vi "PNA_SHEET_DISPLAY.vi"(4 "Mode":i32(ring) items=["OFF", "ON"], 6 "SHEET":i32=1, 8 "error in (no error)":errorcluster, 11 "VISA resource name":refnum<visa-resource-name>) -> (0 "error out":errorcluster, 3 "VISA resource name out":refnum<visa-resource-name>)   [LabVIEW 2018, in "Agilent ENA Series.lvlib"]
doc: "Changes the state of each channel of selected channel to the startup state in the trigger system.\n\nWhen this function is executed for a channel in the idle state, it goes into the initiate state immediately. Then, after measurement is executed once, it goes back to the idle state.\n\nIf this function is executed for a channel that is not in the idle state or for which the continuous initiation mode is enabled, an error occurs."
uses:
  Agilent ENA Series.lvlib
panel:
  out "cmd":string
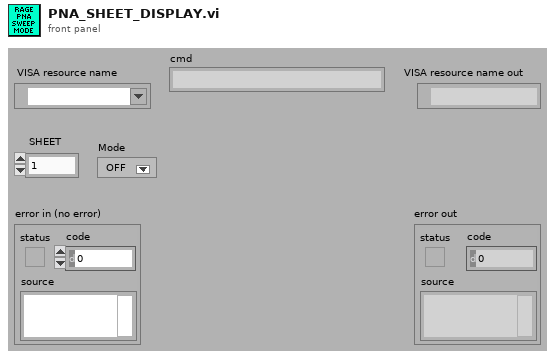
[diagram p1: front panel]
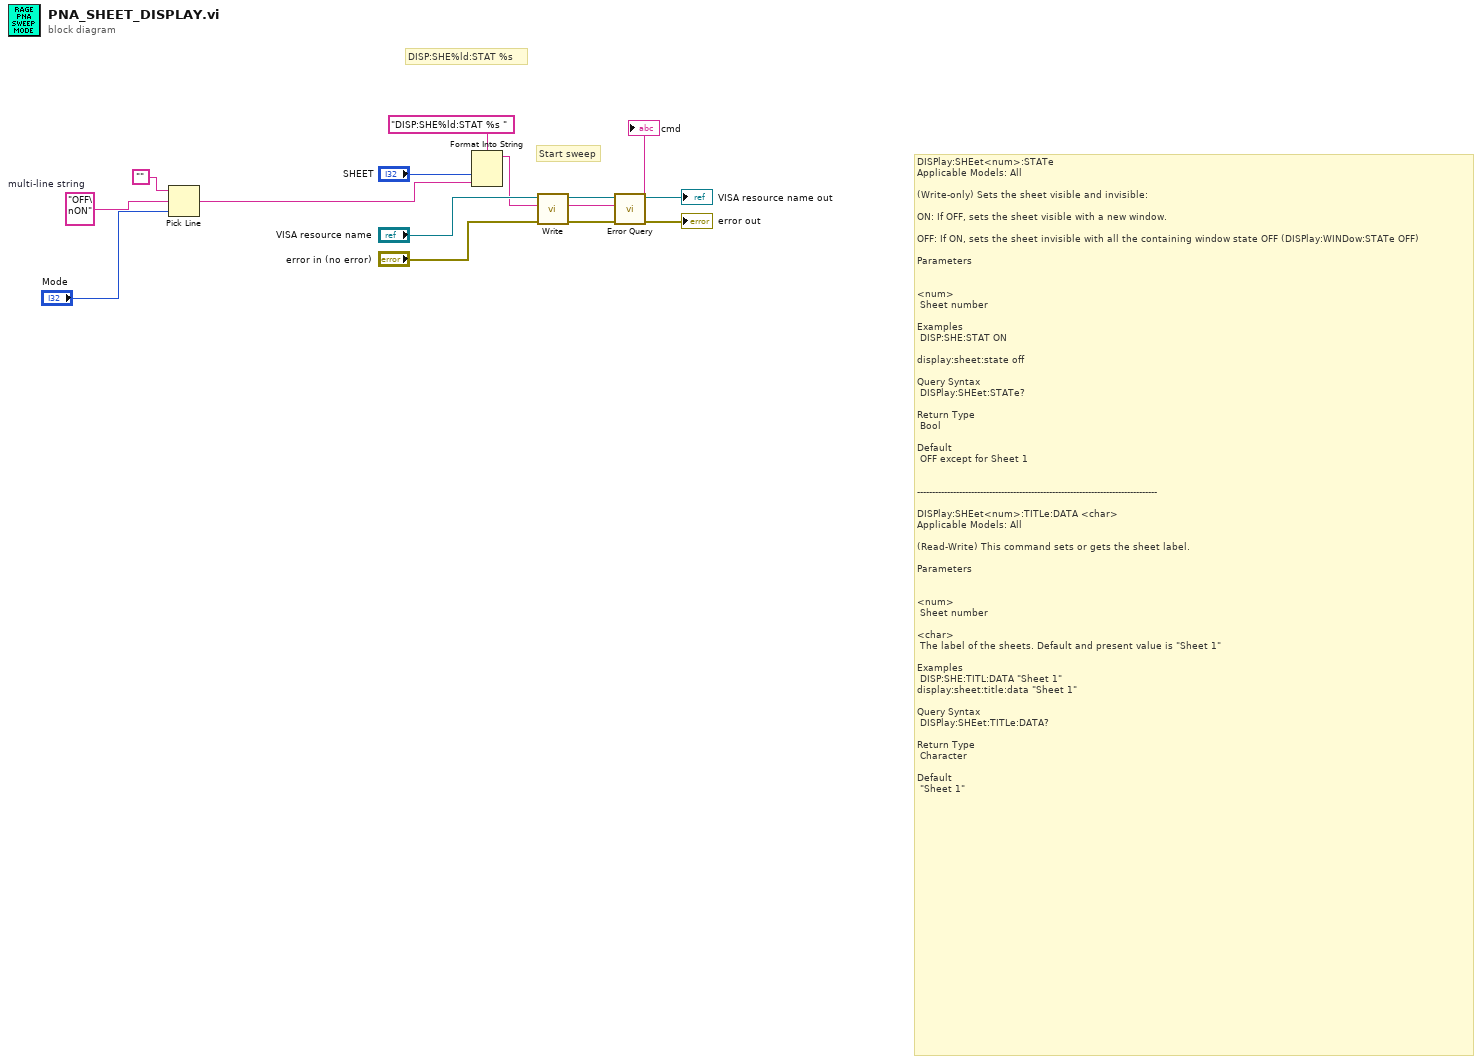
[diagram p0: block diagram]
diagram:
  w4 = "OFF\nON"  # multi-line string
  # "DISP:SHE%ld:STAT %s"
  # "DISPlay:SHEet<num>:STATe\nApplicable Models: All\n\n(Write-only) Sets the sheet visible and invisible:\n\nON: If OFF, sets the sheet visible with a new window.\n\nOFF: If ON, sets the sheet invisible with all the containing window state OFF (DISPlay:WINDow:STATe OFF)\n \nParameters\n  \n \n<num>\n Sheet number\n \nExamples\n DISP:SHE:STAT ON\n\ndisplay:sheet:state off\n \nQuery Syntax\n DISPlay:SHEet:STATe?\n \nReturn Type\n Bool\n \nDefault\n OFF except for Sheet 1\n \n\n--------------------------------------------------------------------------------\n\nDISPlay:SHEet<num>:TITLe:DATA <char>\nApplicable Models: All\n\n(Read-Write) This command sets or gets the sheet label.\n \nParameters\n  \n \n<num>\n Sheet number\n \n<char>\n The label of the sheets. Default and present value is \"Sheet 1\"\n \nExamples\n DISP:SHE:TITL:DATA \"Sheet 1\"\ndisplay:sheet:title:data \"Sheet 1\"\n \nQuery Syntax\n DISPlay:SHEet:TITLe:DATA?\n \nReturn Type\n Character\n \nDefault\n \"Sheet 1\""
  # "Start sweep"
  n1 = Pick Line(string ("")="", multi-line string=w4, line index="Mode") -> (output string=w1:string)
  n2 = Format Into String(format string="DISP:SHE%ld:STAT %s ", "SHEET", w1) -> (resulting string=w9:string)  [unwired: 2 in, 1 out]
  "cmd" <- w9
  n3 = call "Write.vi"("error in (no error)"="error in (no error)", "String ()"=w9, "VISA resource name"="VISA resource name") -> ("error out"=w7:errorcluster, "VISA resource name out"=w8:refnum<visa-resource-name>)  [unwired: 6 in, 1 out]
  n4 = call "Error Query.vi"("error in (no error)"=w7, "VISA resource name"=w8) -> ("error out"=→"error out":errorcluster, "VISA resource name out"=→"VISA resource name out":refnum<visa-resource-name>)  [unwired: 6 in, 2 out]
